vi "ArdnoPumpStepsForRefreshRatio.vi"(10 "ReactorRefreshRatio":dbl, 11 "Desired Refresh Ratio":dbl) -> (3 "Pump steps for the\n desired refresh ratio":dbl)   [LabVIEW 2018, in "Arduino.lvlib"]
uses:
  Arduino.lvlib
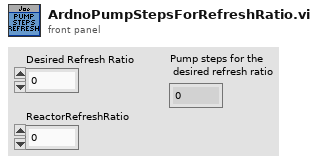
[diagram p1: front panel]
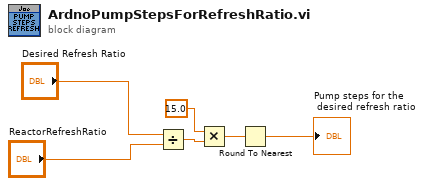
[diagram p0: block diagram]
diagram:
  n1 = Divide(x="Desired Refresh Ratio", y="ReactorRefreshRatio") -> (x/y=w5:dbl)
  n2 = Multiply(x=15.0, y=w5) -> (x*y=w4:dbl)
  n3 = Round To Nearest(number=w4) -> (nearest integer value=→"Pump steps for the\n desired refresh ratio":dbl)
